vi "Retarget Payload.vi"(4 "Payload in":string, 5 "Target Node":u32) -> (7 "Payload out":string)   [LabVIEW 2020, in "Vecto.lvlib" / "TCPMessaging.lvclass"]
uses:
  TCPMessaging.lvclass
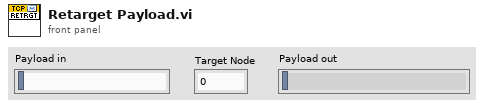
[diagram p1: front panel]
types:
  T1 = enum16{"big-endian, network order", "native, host order", "little-endian"}
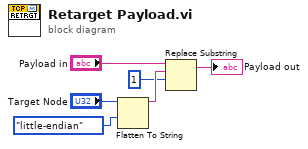
[diagram p0: block diagram]
diagram:
  n1 = Flatten To String(anything="Target Node", byte order (0:big-endian, network order)=T1."little-endian") -> (data string=w3:string)  [unwired: 2 in, 2 out]
  n2 = Replace Substring(3:1 ("offset (0)"), 4:w3, 5:"Payload in") -> (1:→"Payload out":string)  [unwired: 1 in, 1 out]
